vi "Read Digital Input.vi"(8 "error in (no error)":errorcluster, 10 "DI Channel":T1, 11 "LINX-AutomationHat in":refnum<class "LINX-AutomationHat.lvclass">) -> (0 "error out":errorcluster, 2 "Value":bool, 3 "LINX-AutomationHat out":refnum<class "LINX-AutomationHat.lvclass">)   [LabVIEW 2020, in "LINX-AutomationHat.lvclass"]
doc: "Reads the automation-hats digital inputs."
uses:
  LINX-AutomationHat.lvclass
  DI Channels.ctl
  LEDs.ctl
  GPIO/LINX GPIO.lvclass
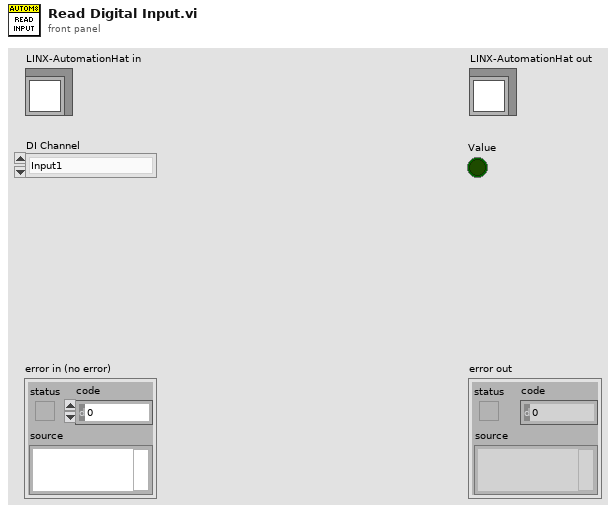
[diagram p1: front panel]
types:
  T1 = typedef "LINX-AutomationHat.lvclass/DI Channels.ctl" = enum16{"Input1", "Input2", "Input3"}
  T2 = typedef "LINX-AutomationHat.lvclass/LEDs.ctl" = enum16{"All", "ADC1", "ADC2", "ADC3", "Output1", "Output2", "Output3", "Relay1NO", "Relay1NC", "Relay2NO", "Relay2NC", "Relay3NO", "Relay3NC", "Input3", "Input2", "Input1", "Warn", "Comms", "Power"}
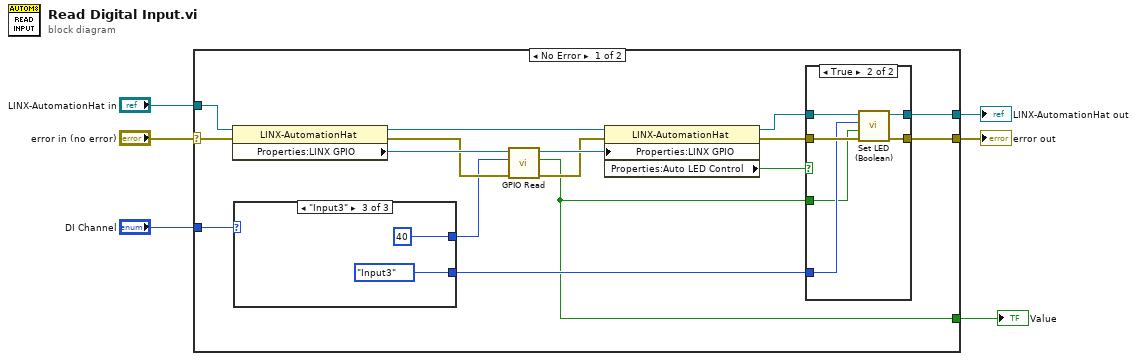
[diagram p0: block diagram]
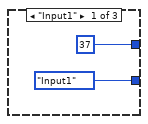
[diagram p3: hidden frame]
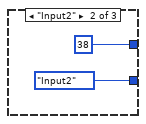
[diagram p4: hidden frame]
diagram:
  n1 = case shown="No Error" "error in (no error)" {
    selector: "error in (no error)" -> [w12 w38]
    tunnel: [w19 w38] -> w5
    tunnel: [w22 w37] -> w3
    tunnel: "LINX-AutomationHat in" -> [w18 w37]
    tunnel: "DI Channel" -> [w11 _]
    tunnel: [w7 _] -> w1
    frame No Error {
      n2 = property class="LINX-AutomationHat"(reference=w18, error in=w12) -> (reference out=w17:refnum<class "LINX-AutomationHat.lvclass">, error out=w14:errorcluster, "Properties:LINX GPIO"=w16:refnum<class "LINX GPIO.lvclass">)
      n3 = case shown="\"Input3\"" w11 {
        tunnel: [u8 37 ("DO Channel") u8 38 ("DO Channel") u8 40 ("DO Channel")] -> w10
        tunnel: [LEDs."Input1" ("LED Selector") LEDs."Input2" ("LED Selector") LEDs."Input3" ("LED Selector")] -> w9
        frame "Input1" {
        }
        frame "Input2" {
        }
        frame "Input3" {
        }
      }
      n4 = call-dynamic "GPIO Read.vi"("error in (no error)"=w14, "DO Channel"=w10, "LINX GPIO in"=w16) -> ("error out"=w13:errorcluster, "Input Value"=w7:bool, "LINX GPIO out"=w15:refnum<class "LINX GPIO.lvclass">)  [unwired: 6 in]
      n5 = property class="LINX-AutomationHat"(reference=w17, error in=w13, "Properties:LINX GPIO"=w15) -> (reference out=w21:refnum<class "LINX-AutomationHat.lvclass">, error out=w20:errorcluster, "Properties:Auto LED Control"=w8:bool)
      n6 = case shown="True" w8 {
        tunnel: [w24 w30] -> w22
        tunnel: w21 -> [w24 w29]
        tunnel: w20 -> [w23 w28]
        tunnel: [w23 w27] -> w19
        tunnel: w9 -> [_ w26]
        tunnel: w7 -> [_ w25]
        frame False {
        }
        frame True {
          n7 = call-dynamic "Set LED (Boolean).vi"("error in (no error)"=w28, "Enable"=w25, "LED Selector"=w26, "LINX-AutomationHat in"=w29) -> ("error out"=w27:errorcluster, "LINX-AutomationHat out"=w30:refnum<class "LINX-AutomationHat.lvclass">)  [unwired: 6 in]
        }
      }
    }
    frame Error {
    }
  }
  "error out" <- w5
  "LINX-AutomationHat out" <- w3
  "Value" <- w1
